vi "Ventilator Control.vi"(2 "error in (no error)":errorcluster, 3 "Ventilator (off)":bool) -> (0 "error out":errorcluster, 1 "Ventilator State":bool)   [LabVIEW 2024]
uses:
  <vilib>/Utility/error.llb/DialogType.ctl
  <vilib>/DAQmx/write.llb/DAQmx Write (Digital Bool 1Line 1Point).vi
  <vilib>/DAQmx/read.llb/DAQmx Read (Digital Bool 1Line 1Point).vi
  <vilib>/DAQmx/create/channels.llb/DAQmx Create Channel (DO-Digital Output).vi
  <vilib>/DAQmx/miscellaneous.llb/DAQmx Fill In Error Info.vi
  <vilib>/DAQmx/create/channels.llb/DAQmx Create Channel (DI-Digital Input).vi
panel:
  in  "Input Line":tag="Dev1/port0/line0"
  in  "Output line":tag="Dev1/port0/line1"
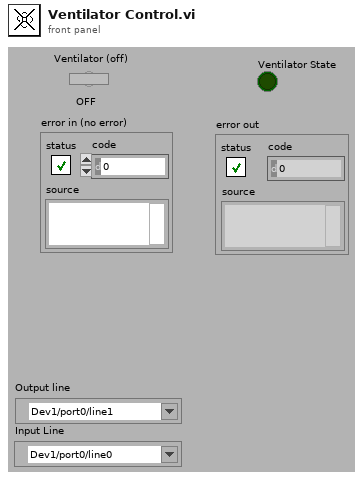
[diagram p1: front panel]
types:
  T1 = typedef "DialogType.ctl" = u16
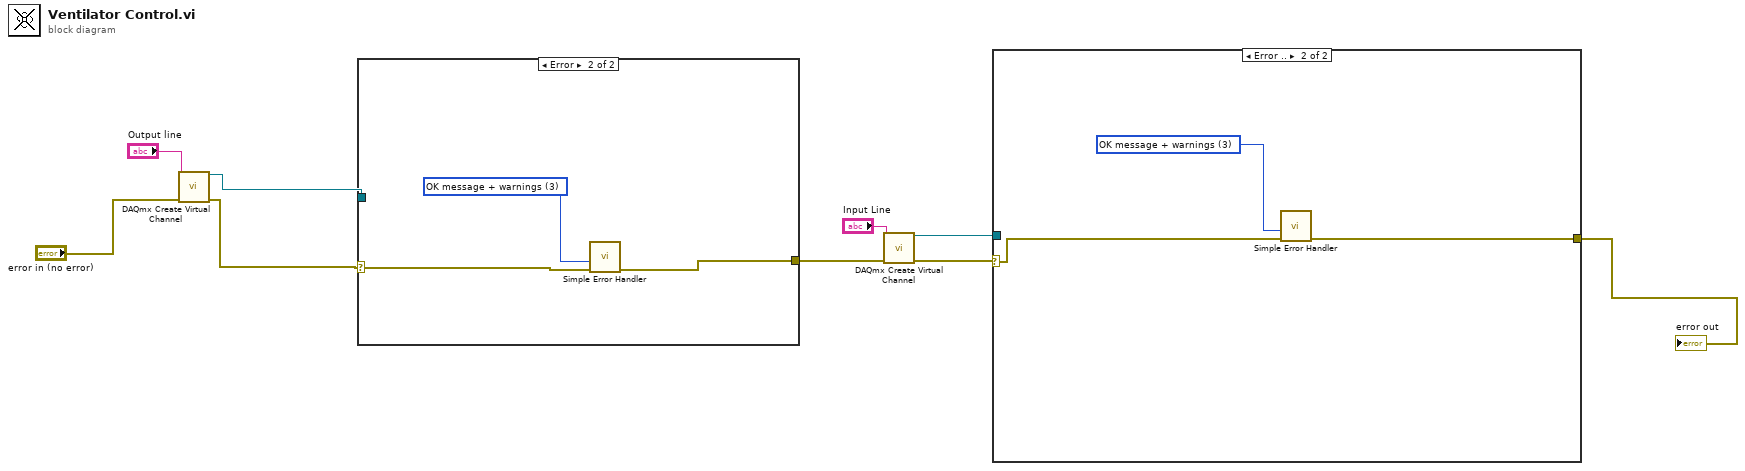
[diagram p0: block diagram]
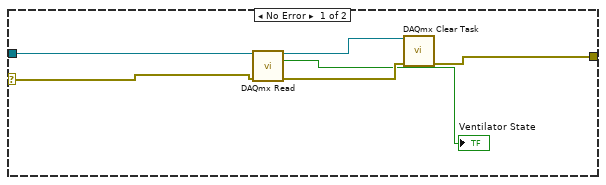
[diagram p2: hidden frame]
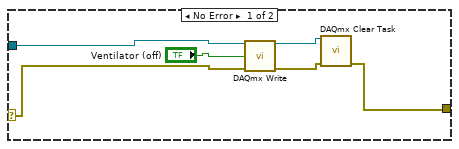
[diagram p3: hidden frame]
diagram:
  n1 = call-poly <vilib>:"DAQmx Create Virtual Channel.vi"("lines"="Output line", "error in"="error in (no error)") -> ("task out"=w9:refnum<k21>, "error out"=w6:errorcluster)  [unwired: 12 in]
  n2 = case shown="Error" w6 {
    selector: w6 -> [w14 w18]
    tunnel: w9 -> [w15 _]
    tunnel: [w11 w17] -> w5
    frame No Error {
      n3 = call-poly <vilib>:"DAQmx Write.vi"("task/channels in"=w15, "data"="Ventilator (off)", "error in"=w14) -> ("task out"=w13:refnum<k21>, "error out"=w12:errorcluster)  [unwired: 10 in, 1 out]
      n4 = call <vilib>:"DAQmx Clear Task.vi"("task in"=w13, "error in"=w12) -> ("error out"=w11:errorcluster)  [unwired: 13 in]
    }
    frame Error {
      w16 = T1 3 items=["no dialog", "OK message", "continue or stop message", "OK message + warnings", "continue/stop + warnings"] ("type of dialog (OK msg:1)")
      n5 = call <vilib>:"Simple Error Handler.vi"("type of dialog (OK msg:1)"=w16, "error in (no error)"=w18) -> ("error out"=w17:errorcluster)  [unwired: 3 in, 4 out]
    }
  }
  n6 = call-poly <vilib>:"DAQmx Create Virtual Channel.vi"("lines"="Input Line", "error in"=w5) -> ("task out"=w3:refnum<k21>, "error out"=w4:errorcluster)  [unwired: 12 in]
  n7 = case shown="Error .." w4 {
    selector: w4 -> [w22 w27]
    tunnel: [w21 w26] -> w2
    tunnel: w3 -> [w20 _]
    frame No Error {
      n8 = call-poly <vilib>:"DAQmx Read.vi"("task/channels in"=w20, "error in"=w22) -> ("task out"=w24:refnum<k21>, "data"=→"Ventilator State":bool, "error out"=w23:errorcluster)  [unwired: 11 in]
      n9 = call <vilib>:"DAQmx Clear Task.vi"("task in"=w24, "error in"=w23) -> ("error out"=w21:errorcluster)  [unwired: 13 in]
    }
    frame Error {
      w25 = T1 3 items=["no dialog", "OK message", "continue or stop message", "OK message + warnings", "continue/stop + warnings"] ("type of dialog (OK msg:1)")
      n10 = call <vilib>:"Simple Error Handler.vi"("type of dialog (OK msg:1)"=w25, "error in (no error)"=w27) -> ("error out"=w26:errorcluster)  [unwired: 3 in, 4 out]
    }
  }
  "error out" <- w2
